vi "FR Load XCL template.vi"(11 "FR measurement":T1={"Measurement frequencies (Hz)"=[1000.0, 10000.0, 1000.0], "Sampling frequency (Hz)"=500000.0, "Signal amplitude (V)"=4.5, "AC-DC settle time (s)"=20.0, "Record length (multiples of period)"=[1000.0, 10000.0, 1000.0], "Measurement template file"=path "", "Row of START keyword"=0, "Row of STOP keyword"=0, "Calculate RMS from samples"=FALSE, "AC-DC warm up time (s)"=300.0, "Measurement template line"=[], "DC meter readings No."=10, "Algorithm"="TWM-WFFT", "Simultaneous measurement"=FALSE, "Recalculate-skip already calculated"=FALSE} {"Record length (multiples of period)" format="%#_3p"; "Sampling frequency (Hz)" format="%#_3p"; "Measurement frequencies (Hz)" format="%#_3p"}) -> (3 "FR measurement out":T1={"Measurement frequencies (Hz)"=[1000.0, 10000.0, 1000.0], "Sampling frequency (Hz)"=500000.0, "Signal amplitude (V)"=4.5, "AC-DC settle time (s)"=20.0, "Record length (multiples of period)"=[1000.0, 10000.0, 1000.0], "Measurement template file"=path "", "Row of START keyword"=0, "Row of STOP keyword"=0, "Calculate RMS from samples"=FALSE, "AC-DC warm up time (s)"=300.0, "Measurement template line"=[], "DC meter readings No."=10, "Algorithm"="TWM-WFFT", "Simultaneous measurement"=FALSE, "Recalculate-skip already calculated"=FALSE} {"Record length (multiples of period)" format="%#_3p"; "Sampling frequency (Hz)" format="%#_3p"; "Measurement frequencies (Hz)" format="%#_3p"})   [LabVIEW 2020]
doc: "Reads values from measurement template in excell spreadsheet."
uses:
  <vilib>/Utility/NIReport.llb/Report Type.ctl
  <vilib>/Utility/error.llb/DialogType.ctl
  <vilib>/addons/_office/excel.llb/Excel Get Data ([str]).vi
  <vilib>/Utility/NIReport.llb/NI_report.lvclass
  <vilib>/addons/_office/NI_ReportGenerationToolkit.lvlib
  <vilib>/Utility/NIReport.llb/NI_ReportGenerationCore.lvlib
  <vilib>/Utility/NIReport.llb/Excel/NI_Excel.lvclass
  FR Measurement/Type definitions/FR measuement.ctl
panel:
  out "Stop row":i32
  out "Start row":i32
  out "excell template content":string[][](array[string])
  out "error out":errorcluster
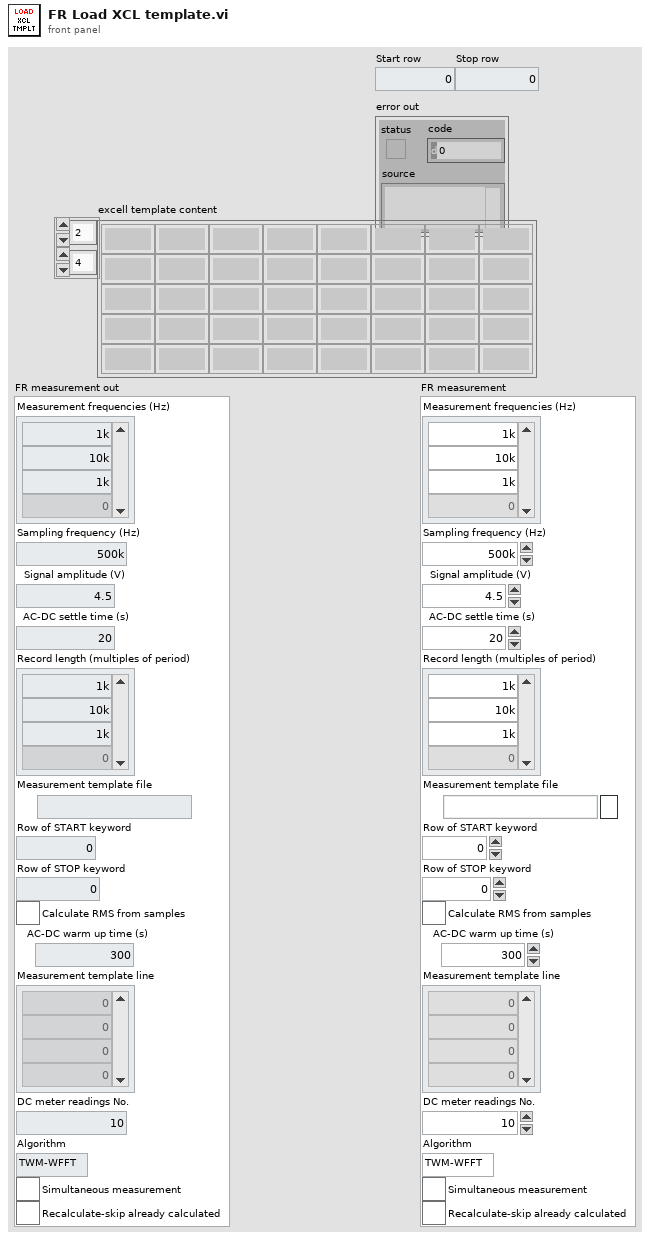
[diagram p1: front panel]
types:
  T1 = typedef "FR measuement.ctl" = cluster{"Measurement frequencies (Hz)":dbl[], "Sampling frequency (Hz)":dbl, "Signal amplitude (V)":dbl, "AC-DC settle time (s)":dbl, "Record length (multiples of period)":dbl[], "Measurement template file":path, "Row of START keyword":i32, "Row of STOP keyword":i32, "Calculate RMS from samples":bool, "AC-DC warm up time (s)":dbl, "Measurement template line":i32[], "DC meter readings No.":i32, "Algorithm":string, "Simultaneous measurement":bool, "Recalculate-skip already calculated":bool}
  T2 = enum16{"maximized", "minimized", "normal", "no change"}
  T3 = typedef "NI_ReportGenerationCore.lvlib/Report Type.ctl" = enum16{"HTML", "Word", "Excel"}
  T4 = typedef "Common properties.ctl" = cluster{"Measurement status ref":refnum<vi>, "TWM Status ref":refnum<vi>, "Abort ref":refnum<vi>, "Skip waiting ref":refnum<vi>, "GNU Octave path":path, "TWM+QWTB path":path, "lvlib path":path, "TWM pipe":string}
  T5 = typedef "AC Source.ctl" = cluster{"AC Source type":T6, "VISA":refnum<visa-resource-name>, "Ref. clock (Hz)":dbl, "status ref":refnum<vi>}
  T6 = typedef "AC Source type.ctl" = enum16{"Fluke 5XXX calibrator", "Tektronix AFG3000 series", "dummy"}
  T7 = typedef "DC meter.ctl" = cluster{"DC meter type":T8, "DC meter VISA":refnum<visa-resource-name>, "NPLC":i32, "status ref":refnum<vi>}
  T8 = typedef "DC meter type.ctl" = enum16{"H/A/K 3458", "Fluke 8508A", "dummy", "Keithley 2182"}
  T9 = typedef "CE measurement.ctl" = cluster{"Signal frequencies (Hz)":dbl[], "Signal amplitudes (V)":dbl[], "Sampling frequencies (Hz)":dbl[], "Record lengths (multiples of periods)":dbl[], "TWM data directories":string[], "Calculate RMS from samples":bool, "RMS algorithm":string, "Settle down after AC source change (s)":dbl}
  T10 = typedef "FR template.ctl" = cluster{"Keywords column":i32, "Sig. freq. column":i32, "Rec. len. column":i32, "Meas. points. row min to read":i32, "Meas. points. row max to read":i32, "Properties column":i32, "Properties row start":i32, "Properties row end":i32, "Keyword START regexp":string, "Keyword STOP regexp":string, "HW data column":i32, "HW data row start":i32, "HW data row end":i32, "TIme and date column start":i32, "Digitizer value column start ":i32, "DC mean column start ":i32, "DC readings column start":i32}
  T11 = cluster{"Common properties":T4, "AC Source":T5, "DC meter":T7, "CE measurement":T9, "FR measurement":T1, "FR template":T10}
  T12 = typedef "DialogType.ctl" = u16
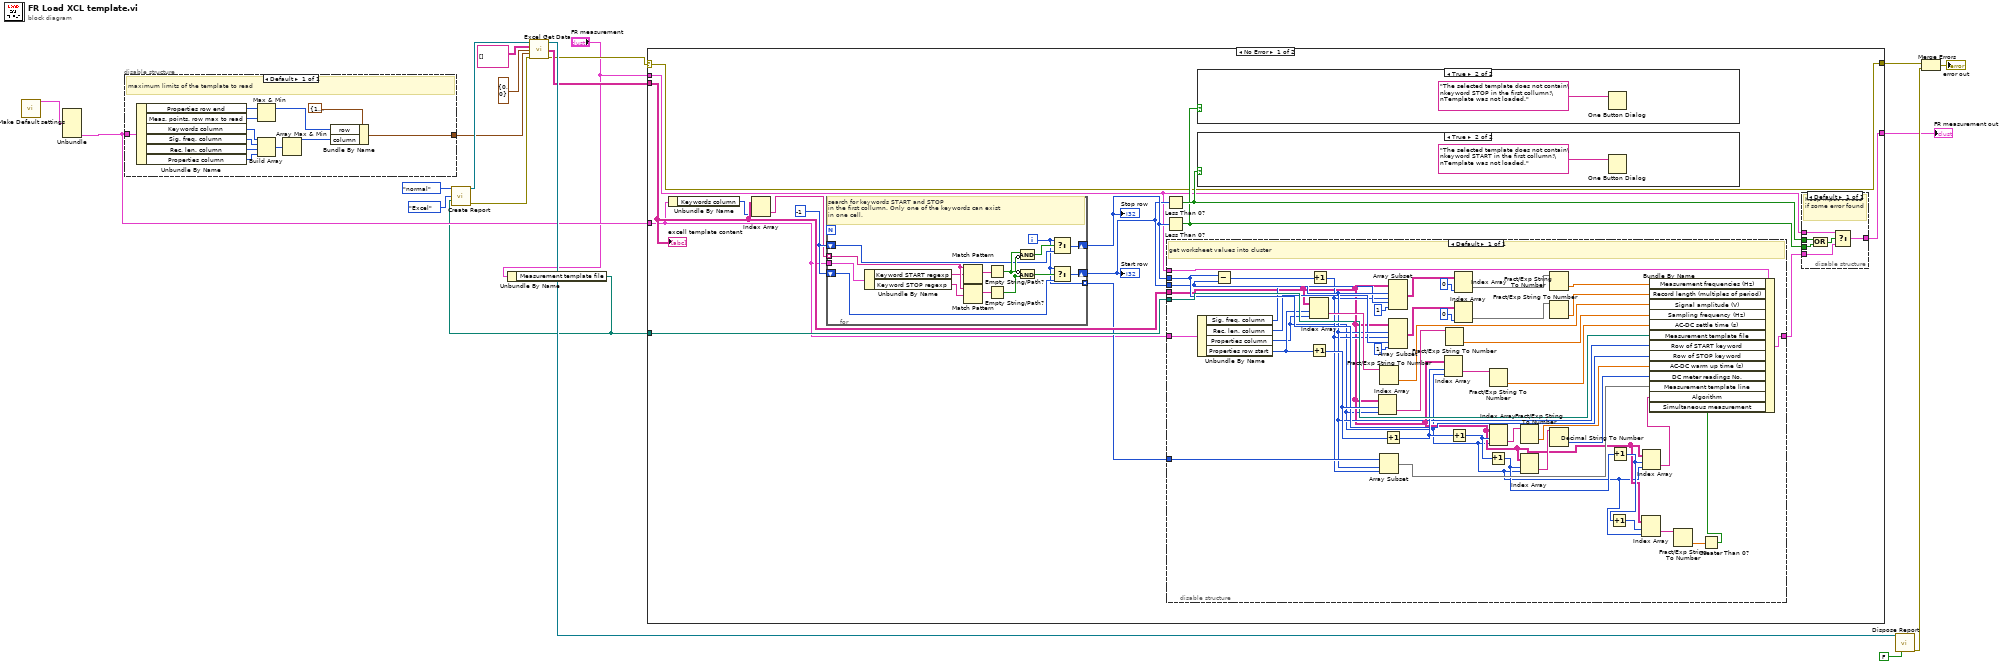
[diagram p0: block diagram]
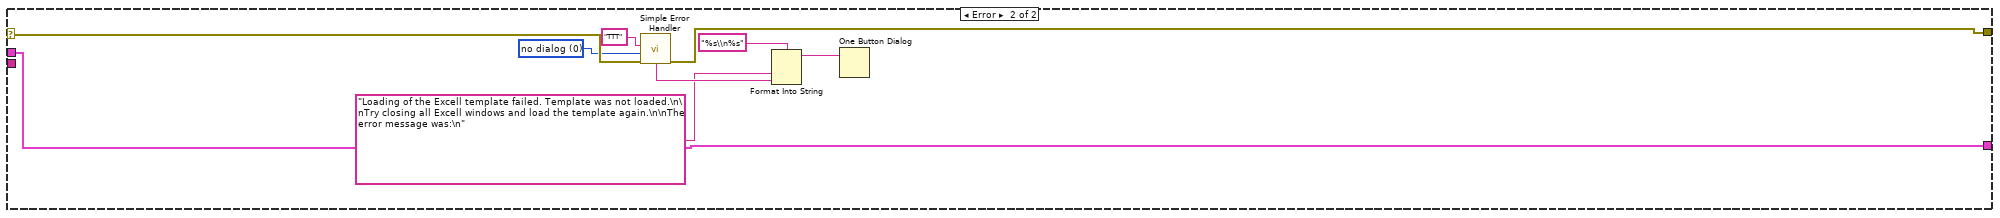
[diagram p4: hidden frame]
diagram:
  n1 = call "Make Default settings.vi"() -> ("All TD"=w4:T11)  [unwired: 11 in]
  n2 = Unbundle(w4) -> ("FR template"=w3:T10)  [unwired: 5 out]
  n3 = disable-structure shown="Default" {
    disable-tunnel: w3 -> [w31]
    disable-tunnel: [w29] -> w6
    frame Enabled {
      # "maximum limits of the template to read"
      n4 = Unbundle By Name(w31) -> ("Properties row end"=w22:i32, "Meas. points. row max to read"=w21:i32, "Keywords column"=w28:i32, "Sig. freq. column"=w27:i32, "Rec. len. column"=w26:i32, "Properties column"=w25:i32)
      n5 = Max & Min(x=w22, y=w21) -> (max(x,y)=w20:i32)  [unwired: 1 out]
      n6 = Build Array(w28, w27, w26, w25) -> (w24:i32[])
      n7 = Array Max & Min(array=w24) -> (max value=w23:i32)  [unwired: 3 out]
      n8 = Bundle By Name(cluster=cluster{"row":i32, "column":i32} {"row"=100000, "column"=7} ("end (-1, -1)"), "row"=w20, "column"=w23) -> (w29:cluster{"row":i32, "column":i32})
    }
  }
  n9 = Unbundle By Name("FR measurement") -> ("Measurement template file"=w2:path)
  n10 = call <vilib>:"Create Report.vi"("window state (normal)"=T2."normal", "report type"=Report_Type."Excel", "template (empty)"=w2) -> ("report out"=w19:refnum<class "NI_report.lvclass">, "error out"=w18:errorcluster)  [unwired: 11 in]
  n11 = call-poly <vilib>:"Excel Get Data.vi"("report in"=w19, "data type"=string[][] [], "start (-1, -1)"=cluster{"row":i32, "column":i32} {"row"=0, "column"=0}, "end (-1, -1)"=w6, "error in (no error)"=w18) -> ("report out"=w17:refnum<class "NI_report.lvclass">, "data"=w13:string[][], "error out"=w10:errorcluster)  [unwired: 8 in]
  n12 = case shown="No Error" w10 {
    selector: w10 -> [w35 w122]
    tunnel: w13 -> [w42 _]
    tunnel: [w38 w123] -> w5
    tunnel: "FR measurement" -> [w37 w123]
    tunnel: w2 -> [w36 _]
    tunnel: [w35 w119] -> w9
    tunnel: w3 -> [w33 _]
    frame No Error {
      w46 = -1
      n13 = Unbundle By Name(w33) -> ("Keywords column"=w32:i32)
      n14 = Index Array(array=w42, index (col)=w32) -> (element=w45:string[])  [unwired: 1 in]
      n15 = for {
        tunnel: w45 -> [w114] mode=indexing
        shift-right: [w110] -> w43
        shift-left: w46 -> [w104]
        shift-right: [w106] -> w44
        shift-left: w46 -> [w105]
        tunnel: [w103] -> w34 mode=indexing
        tunnel: w33 -> [w102]
        i -> [w103]
        # "search for keywords START and STOP\nin the first collumn. Only one of the keywords can exist\nin one cell."
        n16 = Unbundle By Name(w102) -> ("Keyword START regexp"=w101:string, "Keyword STOP regexp"=w100:string)
        n17 = Match Pattern(string=w114, regular expression=w101) -> (match substring=w113:string)  [unwired: 1 in, 3 out]
        n18 = Match Pattern(string=w114, regular expression=w100) -> (match substring=w112:string)  [unwired: 1 in, 3 out]
        n19 = Empty String/Path?(string/path=w113) -> (empty?=w109:bool)
        n20 = Empty String/Path?(string/path=w112) -> (empty?=w108:bool)
        n21 = Compound Arithmetic op=AND(w109, invert w108) -> (w107:bool)
        n22 = Compound Arithmetic op=AND(invert w109, w108) -> (w111:bool)
        n23 = Select(t=w103, s=w107, f=w105) -> (s? t:f=w106:i32)
        n24 = Select(t=w103, s=w111, f=w104) -> (s? t:f=w110:i32)
      }
      "Start row" <- w43
      "Stop row" <- w44
      n25 = Less Than 0?(x=w43) -> (x < 0?=w41:bool)
      n26 = Less Than 0?(x=w44) -> (x < 0?=w40:bool)
      n27 = disable-structure shown="Default" {
        disable-tunnel: w44 -> [w74]
        disable-tunnel: w43 -> [w71]
        disable-tunnel: w37 -> [w97]
        disable-tunnel: w42 -> [w57]
        disable-tunnel: [w91] -> w39
        disable-tunnel: w36 -> [w78]
        disable-tunnel: w34 -> [w73]
        disable-tunnel: w33 -> [w66]
        frame Enabled {
          # "get worksheet values into cluster"
          n28 = Unbundle By Name(w66) -> ("Sig. freq. column"=w65:i32, "Rec. len. column"=w64:i32, "Properties column"=w54:i32, "Properties row start"=w63:i32)
          n29 = Subtract(x=w74, y=w71) -> (x-y=w72:i32)
          n30 = Index Array(array=w57, index (row)=w63, index (col)=w54) -> (element=w85:string)
          n31 = Increment(x=w63) -> (x+1=w80:i32)
          n32 = Increment(x=w72) -> (x+1=w60:i32)
          n33 = Index Array(array=w57, index (row)=w80, index (col)=w54) -> (element=w83:string)
          n34 = Fract/Exp String To Number(string=w85) -> (number=w84:dbl)  [unwired: 3 in, 1 out]
          n35 = Array Subset(array=w73, index=w71, length=w60) -> (w70:i32[])
          n36 = Increment(x=w80) -> (x+1=w76:i32)
          n37 = Array Subset(array=w57, index (row)=w71, length (row)=w60, index (col)=w65, length (col)=1 ("length")) -> (w95:string[][])
          n38 = Array Subset(array=w57, index (row)=w71, length (row)=w60, index (col)=w64, length (col)=1 ("length")) -> (w88:string[][])
          n39 = Index Array(array=w57, index (row)=w76, index (col)=w54) -> (element=w81:string)
          n40 = Fract/Exp String To Number(string=w83) -> (number=w82:dbl)  [unwired: 3 in, 1 out]
          n41 = Increment(x=w76) -> (x+1=w68:i32)
          n42 = Index Array(array=w95, index (col)=0 ("index (row)")) -> (element=w93:string[])  [unwired: 1 in]
          n43 = Index Array(array=w88, index (col)=0 ("index (row)")) -> (element=w90:string[])  [unwired: 1 in]
          n44 = Increment(x=w68) -> (x+1=w62:i32)
          n45 = Fract/Exp String To Number(string=w81) -> (number=w79:dbl)  [unwired: 3 in, 1 out]
          n46 = Index Array(array=w57, index (row)=w68, index (col)=w54) -> (element=w77:string)
          n47 = Fract/Exp String To Number(string=w77) -> (number=w75:dbl)  [unwired: 3 in, 1 out]
          n48 = Index Array(array=w57, index (row)=w62, index (col)=w54) -> (element=w69:string)
          n49 = Fract/Exp String To Number(string=w93) -> (number=w92:dbl[])  [unwired: 3 in, 1 out]
          n50 = Fract/Exp String To Number(string=w90) -> (number=w86:dbl[])  [unwired: 3 in, 1 out]
          n51 = Decimal String To Number(string=w69) -> (number=w67:i32)  [unwired: 2 in, 1 out]
          n52 = Increment(x=w62) -> (x+1=w58:i32)
          n53 = Increment(x=w58) -> (x+1=w59:i32)
          n54 = Index Array(array=w57, index (row)=w59, index (col)=w54) -> (element=w56:string)
          n55 = Index Array(array=w57, index (row)=w58, index (col)=w54) -> (element=w61:string)
          n56 = Fract/Exp String To Number(string=w56) -> (number=w55:dbl)  [unwired: 3 in, 1 out]
          n57 = Greater Than 0?(x=w55) -> (x > 0?=w53:bool)
          n58 = Bundle By Name(cluster=w97, "Measurement frequencies (Hz)"=w92, "Record length (multiples of period)"=w86, "Signal amplitude (V)"=w84, "Sampling frequency (Hz)"=w82, "AC-DC settle time (s)"=w79, "Measurement template file"=w78, "Row of START keyword"=w71, "Row of STOP keyword"=w74, "AC-DC warm up time (s)"=w75, "DC meter readings No."=w67, "Measurement template line"=w70, "Algorithm"=w61, "Simultaneous measurement"=w53) -> (w91:T1)
        }
      }
      n59 = case shown="True" w40 {
        frame False {
        }
        frame True {
          n60 = One Button Dialog(message="The selected template does not contain\nkeyword STOP in the first collumn!\nTemplate was not loaded.") -> ()  [unwired: 1 in, 1 out]
        }
      }
      n61 = case shown="True" w41 {
        frame False {
        }
        frame True {
          n62 = One Button Dialog(message="The selected template does not contain\nkeyword START in the first collumn!\nTemplate was not loaded.") -> ()  [unwired: 1 in, 1 out]
        }
      }
      n63 = disable-structure shown="Default" {
        disable-tunnel: w41 -> [w51]
        disable-tunnel: w40 -> [w50]
        disable-tunnel: w39 -> [w49]
        disable-tunnel: [w48] -> w38
        disable-tunnel: w37 -> [w47]
        frame Enabled {
          # "Keep input values\nif some error found"
          n64 = Compound Arithmetic op=OR(w51, w50) -> (w52:bool)
          n65 = Select(t=w47, s=w52, f=w49) -> (s? t:f=w48:T1)
        }
      }
      "excell template content" <- w42
    }
    frame Error {
      w121 = T12 0 items=["no dialog", "OK message", "continue or stop message", "OK message + warnings", "continue/stop + warnings"] ("type of dialog (OK msg:1)")
      n66 = call <vilib>:"Simple Error Handler.vi"("error source (\" \")"="TTT" ("error source (\" \")"), "type of dialog (OK msg:1)"=w121, "error in (no error)"=w122) -> ("error out"=w119:errorcluster, "message"=w116:string)  [unwired: 2 in, 3 out]
      n67 = Format Into String(format string="%s\\n%s", "Loading of the Excell template failed. Template was not loaded.\n\nTry closing all Excell windows and load the template again.\n\nThe error message was:\n" ("input 1"), w116) -> (resulting string=w117:string)  [unwired: 2 in, 1 out]
      n68 = One Button Dialog(message=w117) -> ()  [unwired: 1 in, 1 out]
    }
  }
  "FR measurement out" <- w5
  n69 = call-dynamic "Dispose Report.vi"("report in"=w17, "close report? (T)"=FALSE) -> ("error out"=w8:errorcluster)  [unwired: 13 in]
  n70 = Merge Errors(w9, w8) -> (→"error out":errorcluster)
